vi "SRV_JPEG Filepath_QR.vi"(1 "QR Code":string, 2 "Dir path for JPEG file":path, 5 "Timestamp String":string) -> (4 "QR Code dup":string, 7 "QR JPEG Filepath":path, 8 "QR Text Filepath":path)   [LabVIEW 2014]
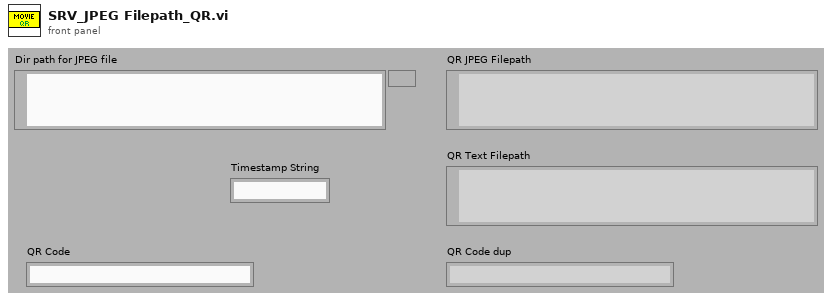
[diagram p1: front panel]
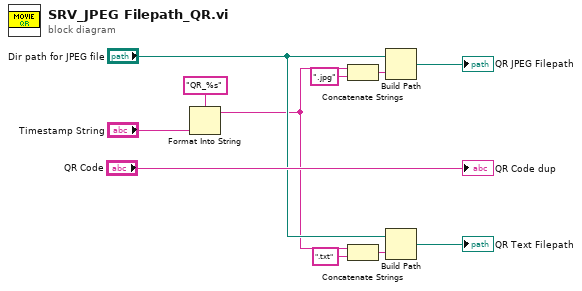
[diagram p0: block diagram]
diagram:
  n1 = Format Into String(format string="QR_%s", "Timestamp String") -> (resulting string=w2:string)  [unwired: 2 in, 1 out]
  n2 = Concatenate Strings(w2, ".jpg" ("string")) -> (w6:string)
  n3 = Concatenate Strings(w2, ".txt" ("string")) -> (w3:string)
  n4 = Build Path(base path="Dir path for JPEG file", name or relative path=w6) -> (appended path=→"QR JPEG Filepath":path)
  n5 = Build Path(base path="Dir path for JPEG file", name or relative path=w3) -> (appended path=→"QR Text Filepath":path)
  "QR Code dup" <- "QR Code"
